vi "Stop Dependency.vi"(8 "error in (no error)":errorcluster, 11 "Dependency in":refnum<class "Dependency.lvclass">) -> (0 "error out":errorcluster, 3 "Dependency out":refnum<class "Dependency.lvclass">)   [LabVIEW 2013, in "Dependency.lvclass"]
uses:
  Dependency.lvclass
  SMO/SMO.lvclass
  Dependency.lvclass/Dependency.ctl
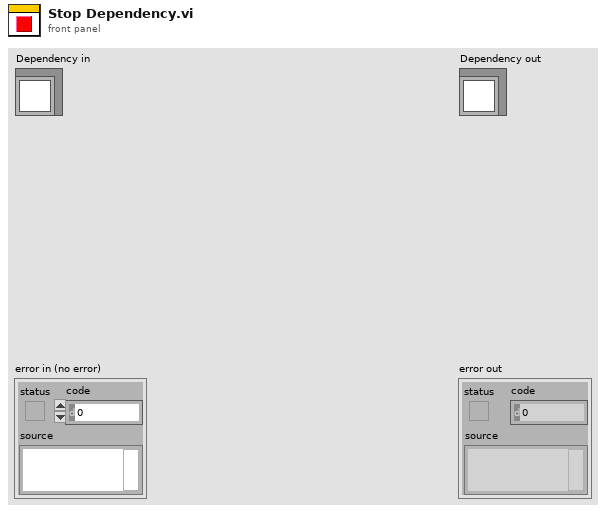
[diagram p1: front panel]
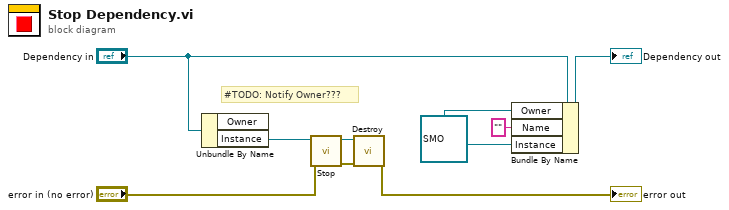
[diagram p0: block diagram]
diagram:
  w2 = refnum<class "SMO.lvclass"> refnum ("Instance")
  # "#TODO: Notify Owner???"
  n1 = Unbundle By Name("Dependency in") -> ("Instance"=w6:refnum<class "SMO.lvclass">)  [unwired: 1 out]
  n2 = call "Stop.vi"("error in (no error)"="error in (no error)", "SMO"=w6) -> ("error out"=w4:errorcluster, "SMO out"=w5:refnum<class "SMO.lvclass">)  [unwired: 8 in]
  n3 = call "Destroy.vi"("error in (no error)"=w4, "SMO"=w5) -> ("error out"=→"error out":errorcluster)  [unwired: 9 in]
  n4 = Bundle By Name(cluster="Dependency in", "Owner"=w2, "Name"="", "Instance"=w2) -> (→"Dependency out":refnum<class "Dependency.lvclass">)
